vi "Create From Variant (Numeric).vi"(8 "error in (no error)":errorcluster, 10 "Variant":variant, 11 "JSON Numeric in":refnum<class "JSON Helper.lvclass">) -> (0 "error out":errorcluster, 3 "JSON Numeric out":refnum<class "JSON Helper.lvclass">)   [LabVIEW 2016, in "JSON Helper.lvclass"]
doc: "Creates a new JSON instance from the given Variant."
uses:
  JSON Helper/JSON Helper.lvclass
  JSON Helper/JSON Helper.lvclass/JSON Helper.ctl
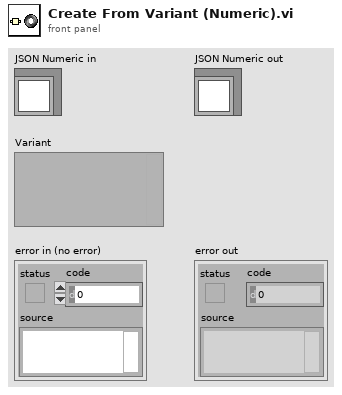
[diagram p1: front panel]
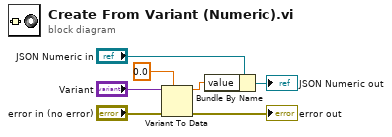
[diagram p0: block diagram]
diagram:
  n1 = Variant To Data(error in="error in (no error)", type=0.0, Variant="Variant") -> (data=w4:dbl, error out=→"error out":errorcluster)
  n2 = Bundle By Name(cluster="JSON Numeric in", "value"=w4) -> (→"JSON Numeric out":refnum<class "JSON Helper.lvclass">)
